vi "Boolean to Display Values.vi"(10 "Offset":i32, 11 "Array":bool[][](array[boolean])) -> (2 "Right":u8[](array[numeric]), 3 "Left":u8[](array[numeric]))   [LabVIEW 2026, in "LED Matrix.lvlib" / "LED Matrix.lvclass"]
uses:
  LED Matrix.lvclass
  LED Matrix.lvclass/LED Matrix.ctl
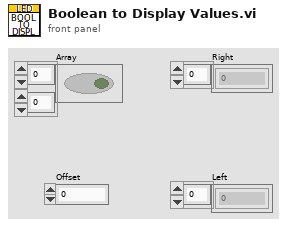
[diagram p1: front panel]
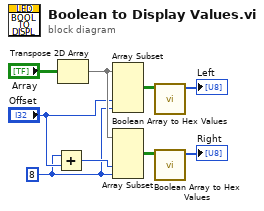
[diagram p0: block diagram]
diagram:
  w6 = 8 ("length")
  n1 = Add(x=w6, y="Offset") -> (x+y=w7:i32)
  n2 = Transpose 2D Array(2D array="Array") -> (transposed array=w9:bool[][])
  n3 = Array Subset(array=w9, index (col)="Offset", length (col)=w6) -> (w3:bool[][])  [unwired: 2 in]
  n4 = Array Subset(array=w9, index (col)=w7, length (col)=w6) -> (w4:bool[][])  [unwired: 2 in]
  n5 = call "Boolean Array to Hex Values.vi"("Array in"=w3) -> ("Array out"=→"Left":u8[])  [unwired: 10 in]
  n6 = call "Boolean Array to Hex Values.vi"("Array in"=w4) -> ("Array out"=→"Right":u8[])  [unwired: 10 in]
